vi "HEX2文本.vi"(10 "读内部参数":string[](array[string])) -> (2 "内部参数(文本)":string[](array[string]))   [LabVIEW 2020]
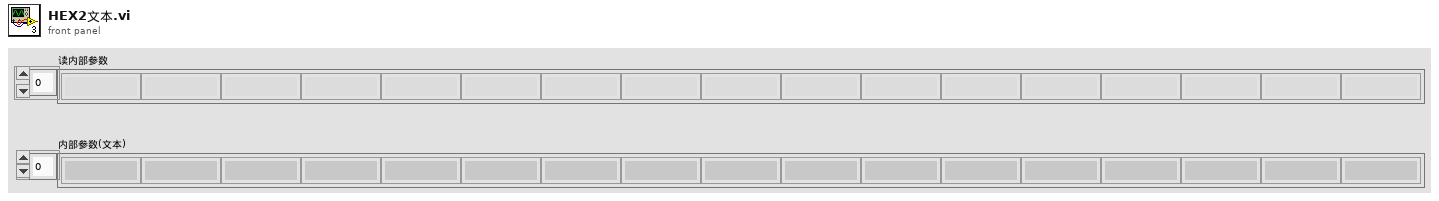
[diagram p1: front panel]
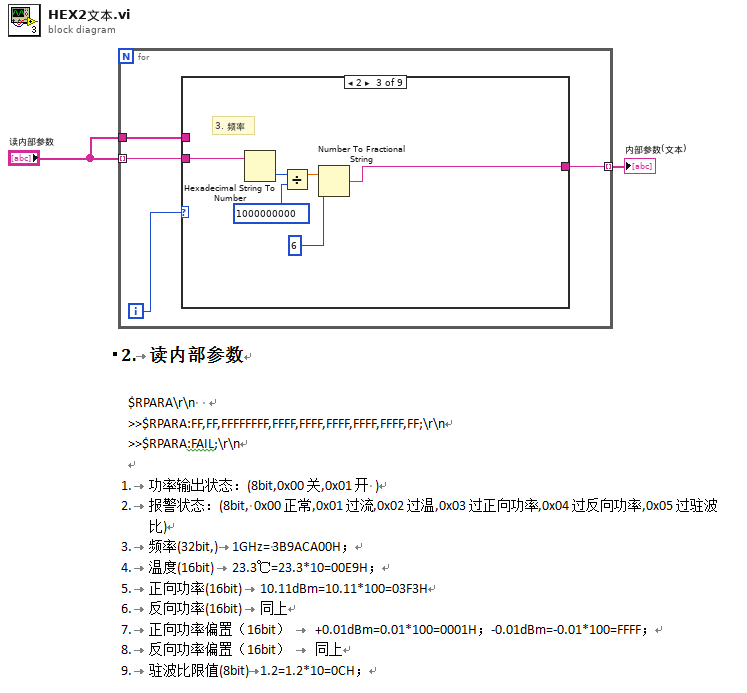
[diagram p0: block diagram]
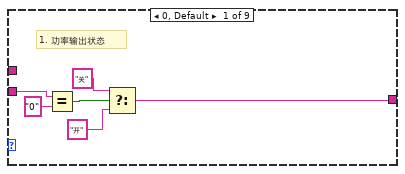
[diagram p2: hidden frame]
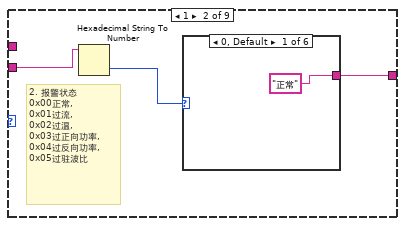
[diagram p3: hidden frame]
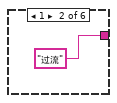
[diagram p4: hidden frame]
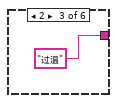
[diagram p5: hidden frame]
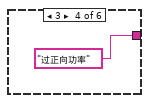
[diagram p6: hidden frame]
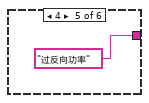
[diagram p7: hidden frame]
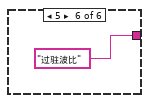
[diagram p8: hidden frame]
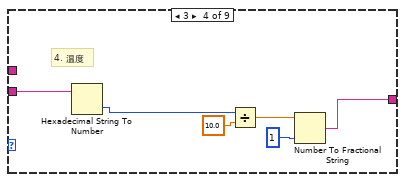
[diagram p9: hidden frame]
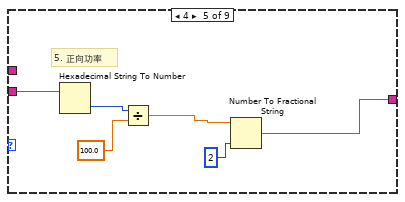
[diagram p10: hidden frame]
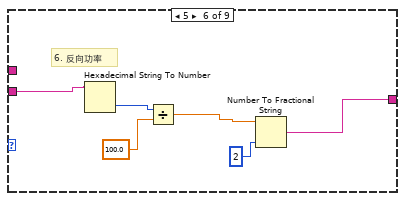
[diagram p11: hidden frame]
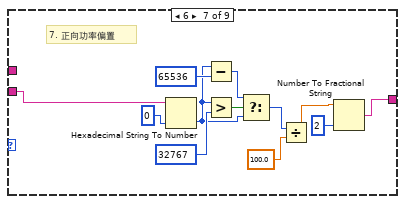
[diagram p12: hidden frame]
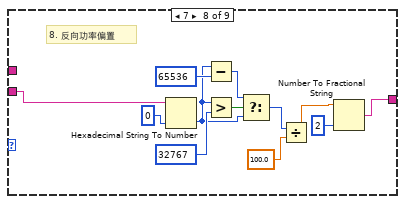
[diagram p13: hidden frame]
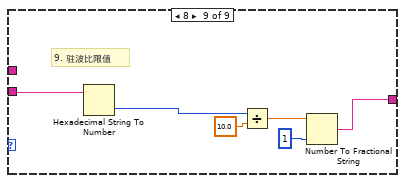
[diagram p14: hidden frame]
diagram:
  n1 = for {
    tunnel: "读内部参数" -> [w5] mode=indexing
    tunnel: [w4] -> w2 mode=indexing
    tunnel: "读内部参数" -> [w3]
    i -> [w6]
    n2 = case shown="2" w6 {
      tunnel: w5 -> [w12 w15 w27 w33 w39 w41 w51 w63 w72]
      tunnel: [w7 w13 w25 w29 w34 w40 w46 w58 w71] -> w4
      tunnel: w3 -> [_ _ _ _ _ _ _ _ _]
      frame 0, Default {
        # "1.\t功率输出状态"
        n3 = Equal?(x=w12, y="0") -> (x = y?=w10:bool)
        n4 = Select(t="关" ("y"), s=w10, f="开" ("y")) -> (s? t:f=w7:string)
      }
      frame 1 {
        # "2.\t报警状态\n0x00正常,\n0x01过流,\n0x02过温,\n0x03过正向功率,\n0x04过反向功率,\n0x05过驻波比"
        n5 = Hexadecimal String To Number(string=w15) -> (number=w14:u32)  [unwired: 2 in, 1 out]
        n6 = case shown="0, Default" w14 {
          tunnel: ["正常" "过流" "过温" "过正向功率" "过反向功率" "过驻波比"] -> w13
          frame 0, Default {
          }
          frame 1 {
          }
          frame 2 {
          }
          frame 3 {
          }
          frame 4 {
          }
          frame 5 {
          }
        }
      }
      frame 2 {
        # "3.\t频率"
        n7 = Hexadecimal String To Number(string=w27) -> (number=w26:u32)  [unwired: 2 in, 1 out]
        n8 = Divide(x=w26, y=u32 1000000000) -> (x/y=w24:dbl)
        n9 = Number To Fractional String(number=w24, precision (6)=i16 6) -> (F-format string=w25:string)  [unwired: 2 in]
      }
      frame 3 {
        # "4.\t温度"
        n10 = Hexadecimal String To Number(string=w33) -> (number=w28:u32)  [unwired: 2 in, 1 out]
        n11 = Divide(x=w28, y=10.0) -> (x/y=w31:dbl)
        n12 = Number To Fractional String(number=w31, precision (6)=i16 1 ("精度(6)")) -> (F-format string=w29:string)  [unwired: 2 in]
      }
      frame 4 {
        # "5.\t正向功率"
        n13 = Hexadecimal String To Number(string=w39) -> (number=w37:u32)  [unwired: 2 in, 1 out]
        n14 = Divide(x=w37, y=100.0) -> (x/y=w35:dbl)
        n15 = Number To Fractional String(number=w35, precision (6)=i16 2 ("精度(6)")) -> (F-format string=w34:string)  [unwired: 2 in]
      }
      frame 5 {
        # "6.\t反向功率"
        n16 = Hexadecimal String To Number(string=w41) -> (number=w44:u32)  [unwired: 2 in, 1 out]
        n17 = Divide(x=w44, y=100.0) -> (x/y=w42:dbl)
        n18 = Number To Fractional String(number=w42, precision (6)=i16 2 ("精度(6)")) -> (F-format string=w40:string)  [unwired: 2 in]
      }
      frame 6 {
        # "7.\t正向功率偏置"
        n19 = Hexadecimal String To Number(string=w51, default (0uL)=0 ("default (0 U32)")) -> (number=w52:i32)  [unwired: 1 in, 1 out]
        n20 = Subtract(x=w52, y=65536) -> (x-y=w54:i32)
        n21 = Greater?(x=w52, y=32767) -> (0:w53:bool)
        n22 = Select(t=w54, s=w53, f=w52) -> (s? t:f=w50:i32)
        n23 = Divide(x=w50, y=100.0) -> (x/y=w48:dbl)
        n24 = Number To Fractional String(number=w48, precision (6)=i16 2) -> (F-format string=w46:string)  [unwired: 2 in]
      }
      frame 7 {
        # "8.\t反向功率偏置"
        n25 = Hexadecimal String To Number(string=w63, default (0uL)=0 ("default (0 U32)")) -> (number=w64:i32)  [unwired: 1 in, 1 out]
        n26 = Subtract(x=w64, y=65536) -> (x-y=w66:i32)
        n27 = Greater?(x=w64, y=32767) -> (0:w65:bool)
        n28 = Select(t=w66, s=w65, f=w64) -> (s? t:f=w62:i32)
        n29 = Divide(x=w62, y=100.0) -> (x/y=w60:dbl)
        n30 = Number To Fractional String(number=w60, precision (6)=i16 2) -> (F-format string=w58:string)  [unwired: 2 in]
      }
      frame 8 {
        # "9.\t驻波比限值"
        n31 = Hexadecimal String To Number(string=w72) -> (number=w70:u32)  [unwired: 2 in, 1 out]
        n32 = Divide(x=w70, y=10.0) -> (x/y=w74:dbl)
        n33 = Number To Fractional String(number=w74, precision (6)=i16 1 ("精度(6)")) -> (F-format string=w71:string)  [unwired: 2 in]
      }
    }
  }
  "内部参数(文本)" <- w2
